vi "PicoHandsOnExample.vi"() -> ()   [LabVIEW 2020]
uses:
  Public/DigIns.ctl
  Public/AnaIns.ctl
  Public/DigOuts.ctl
  <vilib>/CTI/CTI Visa Drivers/CTI-Visa/Identity.ctl
  Public/AOs.ctl
  Public/PWMSettings.ctl
  80566379-07e7-49b1-baf3-c7dff9318c60.vi
  HandsOnPi2040.lvlib
  <vilib>/CTI/CTI Visa Drivers/CTI-Visa/CTI-Visa.lvlib
panel:
  in  "Frequency":sgl(slide) scale=10.0..500000.0
  in  "Duty":sgl(slide) scale=0.0..1.0
  out "Identity":T1
  out "LoopIndex":i32
  in  "Digital Output":T2=enum."DO1 (GPIO2)"
  in  "DOBEEP":bool
  in  "DO4":bool
  in  "DO3":bool
  in  "DO2":bool
  out "AnInValue":u16(graph)
  in  "Analog Input":T3=enum."AI1 (GPIO26)"
  out "DIStatus":bool
  in  "Digital Input":T4=enum."DI1 (GPIO7)"
  out "DOStatus":bool
  in  "DO1":bool
  in  "VISA resource":refnum<visa-resource-name>="COM3"
  out "error out":errorcluster
  in  "stop":bool
  # "WRITE"
  # "READ"
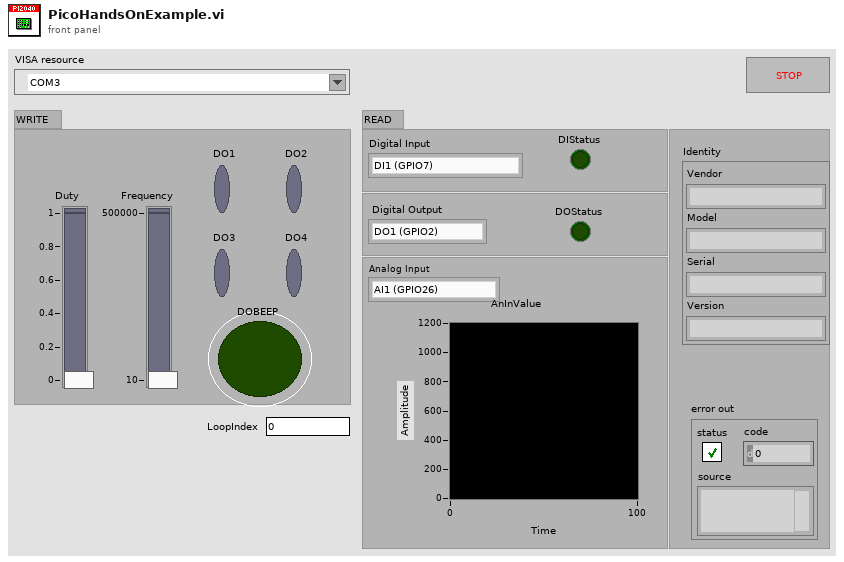
[diagram p1: front panel]
types:
  T1 = typedef "CTI-Visa.lvlib/Identity.ctl" = cluster{"Vendor":string, "Model":string, "Serial":string, "Version":string}
  T2 = typedef "HandsOnPi2040.lvlib/DigOuts.ctl" = enum16{"No DO - Error", "DO1 (GPIO2)", "DO2 (GPIO3)", "DO3 (GPIO4)", "DO4 (GPIO5)", "BEEP (GPIO6)"}
  T3 = typedef "HandsOnPi2040.lvlib/AnaIns.ctl" = enum16{"No AI - Error", "AI1 (GPIO26)", "AI2 (GPIO27)"}
  T4 = typedef "HandsOnPi2040.lvlib/DigIns.ctl" = enum16{"No DI - Error", "DI1 (GPIO7)", "DI2 (GPIO8)", "DI3 (GPIO9)", "DI4 (GPIO10)"}
  T5 = typedef "HandsOnPi2040.lvlib/PWMSettings.ctl" = cluster{"Duty":sgl, "Frequency":sgl}
  T6 = typedef "HandsOnPi2040.lvlib/AOs.ctl" = enum8{"No AO - Error", "AO1 (GPIO28)"}
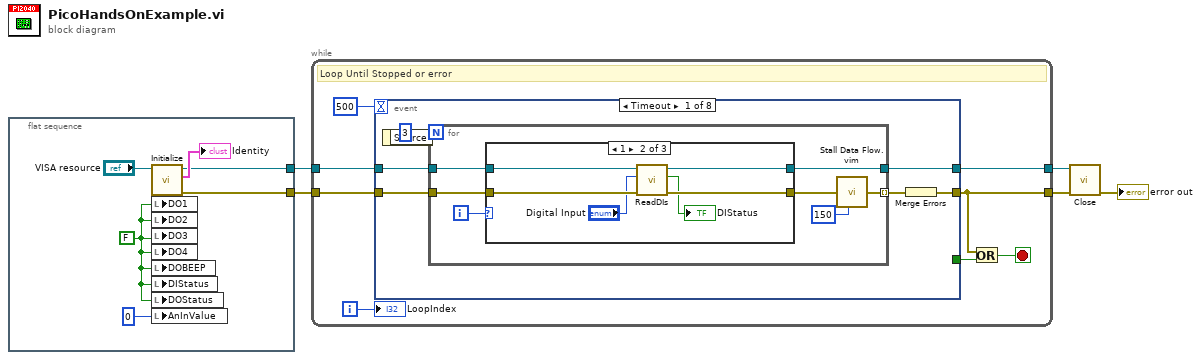
[diagram p0: block diagram]
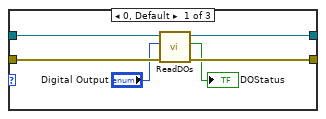
[diagram p2: hidden frame]
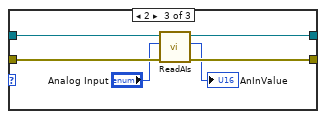
[diagram p3: hidden frame]
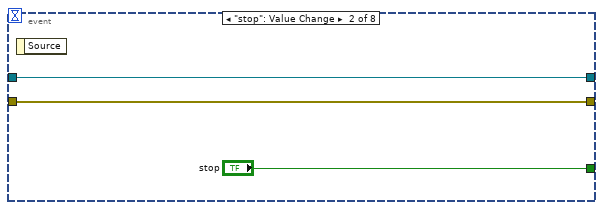
[diagram p4: hidden frame]
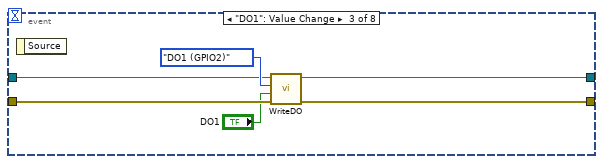
[diagram p5: hidden frame]
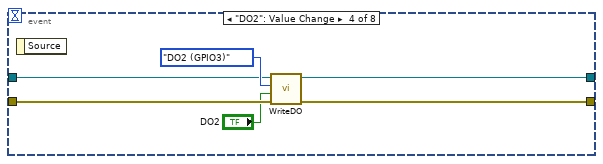
[diagram p6: hidden frame]
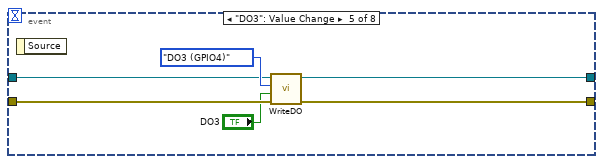
[diagram p7: hidden frame]
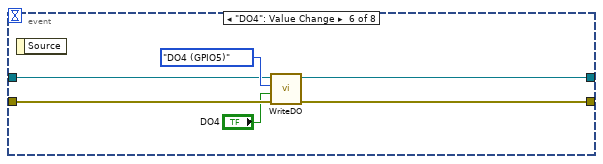
[diagram p8: hidden frame]
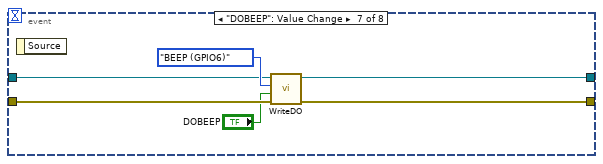
[diagram p9: hidden frame]
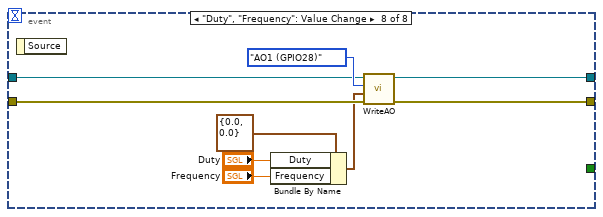
[diagram p10: hidden frame]
diagram:
  n1 = flat-sequence {
    tunnel: [w8] -> w1
    tunnel: [w11] -> w3
    frame #0 {
      w6 = FALSE ("WriteAnOut")
      n2 = call "Initialize.vi"("VISA resource name"="VISA resource") -> ("error out"=w11:errorcluster, "Identity"=→"Identity":T1, "VISA resource name out"=w8:refnum<visa-resource-name>)  [unwired: 8 in]
      n3 = local write "DO1"(w6) -> ()
      n4 = local write "DO2"(w6) -> ()
      n5 = local write "DO3"(w6) -> ()
      n6 = local write "DO4"(w6) -> ()
      n7 = local write "DOBEEP"(w6) -> ()
      n8 = local write "DIStatus"(w6) -> ()
      n9 = local write "DOStatus"(w6) -> ()
      n10 = local write "AnInValue"(u16 0 ("AnInValue")) -> ()
    }
  }
  n11 = while {
    tunnel: [w18] -> w5
    tunnel: w1 -> [w17]
    tunnel: [w16] -> w2
    tunnel: w3 -> [w19]
    i -> [w14]
    stop <- w12 stop-if-true
    # "Loop Until Stopped or error"
    n12 = event shown="[0] Timeout" {
      selector: _ -> [_ _ _ _ _ _ _ _]
      dyn-events: _ -> [_ _ _ _ _ _ _ _]
      timeout: 500 -> [_ _ _ _ _ _ _ _]
      tunnel: [_ "stop" _ _ _ _ _ _] -> w13
      tunnel: [w24 w53 w59 w65 w71 w77 w83 w91] -> w18
      tunnel: w19 -> [w25 w53 w58 w64 w70 w76 w82 w92]
      tunnel: w17 -> [w22 w52 w56 w62 w68 w74 w80 w89]
      tunnel: [w21 w52 w55 w61 w67 w73 w79 w88] -> w16
      event Timeout {
        n13 = event-data() -> ()  [unwired: 1 in, 1 out]
        n14 = for {
          N: 3 -> [_]
          tunnel: w25 -> [w32]
          tunnel: [w30] -> w23 mode=indexing
          tunnel: w22 -> [w28]
          tunnel: [w27] -> w21
          i -> [w29]
          n15 = case shown="1" w29 {
            tunnel: w32 -> [w38 w44 w50]
            tunnel: [w37 w43 w49] -> w31
            tunnel: w28 -> [w36 w42 w48]
            tunnel: [w35 w41 w47] -> w27
            frame 0, Default {
              n16 = call "ReadDOs.vi"("error in"=w38, "Output"="Digital Output", "VISA resource name"=w36) -> ("error out"=w37:errorcluster, "DO Status"=→"DOStatus":bool, "VISA resource name out"=w35:refnum<visa-resource-name>)  [unwired: 6 in]
            }
            frame 1 {
              n17 = call "ReadDIs.vi"("error in"=w44, "Digital Inputs"="Digital Input", "VISA resource name"=w42) -> ("error out"=w43:errorcluster, "DI Status"=→"DIStatus":bool, "VISA resource name out"=w41:refnum<visa-resource-name>)  [unwired: 6 in]
            }
            frame 2 {
              n18 = call "ReadAIs.vi"("error in"=w50, "Analog Inputs"="Analog Input", "VISA resource name"=w48) -> ("error out"=w49:errorcluster, "Value"=→"AnInValue":u16, "VISA resource name out"=w47:refnum<visa-resource-name>)  [unwired: 6 in]
            }
          }
          n19 = call "Stall Data Flow.vim"("value in"=w31, "milliseconds to wait"=u32 150) -> ("value out"=w30:errorcluster)  [unwired: 1 out]
        }
        n20 = Merge Errors(w23) -> (w24:errorcluster)
      }
      event "stop": Value Change {
        n21 = event-data() -> ()  [unwired: 1 in, 1 out]
      }
      event "DO1": Value Change {
        n22 = event-data() -> ()  [unwired: 1 in, 1 out]
        n23 = call "WriteDO.vi"("error in"=w58, "DO Value"="DO1", "Output"=DigOuts."DO1 (GPIO2)" ("Write Digital Output"), "VISA resource name"=w56) -> ("error out"=w59:errorcluster, "VISA resource name out"=w55:refnum<visa-resource-name>)  [unwired: 6 in]
      }
      event "DO2": Value Change {
        n24 = event-data() -> ()  [unwired: 1 in, 1 out]
        n25 = call "WriteDO.vi"("error in"=w64, "DO Value"="DO2", "Output"=DigOuts."DO2 (GPIO3)" ("Write Digital Output"), "VISA resource name"=w62) -> ("error out"=w65:errorcluster, "VISA resource name out"=w61:refnum<visa-resource-name>)  [unwired: 6 in]
      }
      event "DO3": Value Change {
        n26 = event-data() -> ()  [unwired: 1 in, 1 out]
        n27 = call "WriteDO.vi"("error in"=w70, "DO Value"="DO3", "Output"=DigOuts."DO3 (GPIO4)" ("Write Digital Output"), "VISA resource name"=w68) -> ("error out"=w71:errorcluster, "VISA resource name out"=w67:refnum<visa-resource-name>)  [unwired: 6 in]
      }
      event "DO4": Value Change {
        n28 = event-data() -> ()  [unwired: 1 in, 1 out]
        n29 = call "WriteDO.vi"("error in"=w76, "DO Value"="DO4", "Output"=DigOuts."DO4 (GPIO5)" ("Write Digital Output"), "VISA resource name"=w74) -> ("error out"=w77:errorcluster, "VISA resource name out"=w73:refnum<visa-resource-name>)  [unwired: 6 in]
      }
      event "DOBEEP": Value Change {
        n30 = event-data() -> ()  [unwired: 1 in, 1 out]
        n31 = call "WriteDO.vi"("error in"=w82, "DO Value"="DOBEEP", "Output"=DigOuts."BEEP (GPIO6)" ("Write Digital Output"), "VISA resource name"=w80) -> ("error out"=w83:errorcluster, "VISA resource name out"=w79:refnum<visa-resource-name>)  [unwired: 6 in]
      }
      event "Duty", "Frequency": Value Change {
        n32 = event-data() -> ()  [unwired: 1 in, 1 out]
        n33 = Bundle By Name(cluster=T5 {"Duty"=0.0, "Frequency"=0.0} ("PWM Settings"), "Duty"="Duty", "Frequency"="Frequency") -> (w86:T5)
        n34 = call "WriteAO.vi"("error in"=w92, "PWM Settings"=w86, "Analog Output"=AOs."AO1 (GPIO28)", "VISA resource name"=w89) -> ("error out"=w91:errorcluster, "VISA resource name out"=w88:refnum<visa-resource-name>)  [unwired: 6 in]
      }
    }
    n35 = Or(x=w18, y=w13) -> (x .or. y?=w12:bool)
    "LoopIndex" <- w14
  }
  n36 = call "Close.vi"("error in"=w5, "VISA resource name"=w2) -> ("error out"=→"error out":errorcluster)  [unwired: 9 in]
